vi "04Foot.vi"() -> ()   [LabVIEW 2015]
uses:
  <vilib>/Instr/_visa.llb/VISA Configure Serial Port (Serial Instr).vi
  <vilib>/Utility/file.llb/Read Delimited Spreadsheet (DBL).vi
  <vilib>/DAQmx/create/channels.llb/DAQmx Create Channel (DI-Digital Input).vi
  <vilib>/DAQmx/configure/timing.llb/DAQmx Timing (Sample Clock).vi
  <vilib>/Utility/file.llb/Write Delimited Spreadsheet (DBL).vi
  <resource>/objmgr/daqmx.rc
panel:
  out "MPH READ 2":u8
  in  "Tab Control":enum32{"Page 1", "Page 2"}(tab)
  out "NEXT DURATION":dbl format="%#.1f"
  out "NEXT MPH":dbl min=0.0 max=12.0 step=0.1 format="%.1f"
  out "Time Left":dbl format="%#.0f"
  out "ESTOP":bool
  in  "ESTOP RESUME":bool
  out "MPH":dbl min=0.0 max=12.0 step=0.1 format="%.1f"
  out "Foot":dbl
  out "ESTOP2":bool
  out "Report Location":path
  in  "TestScript":path=path "C:/LabVIEW VIs/TRMConsole/FootTime.txt"
  out "Waveform Graph":dbl[](graph)
  out "speed":dbl[](array[numeric])
  out "time":dbl[](array[numeric])
  out "dwell":dbl[](array[numeric])
  out "step":i32
  out "arraysize":i32
  out "x-y":u32
  out "appended path":path
  out "stopping":bool
  out "String":string
  in  "stop":bool
  out "MPH READ":u8
  in  "Serial Port":refnum<visa-resource-name>="COM8"
  in  "lines":tag="DAQMod1/port0"
  out "Enum":T1(ring)
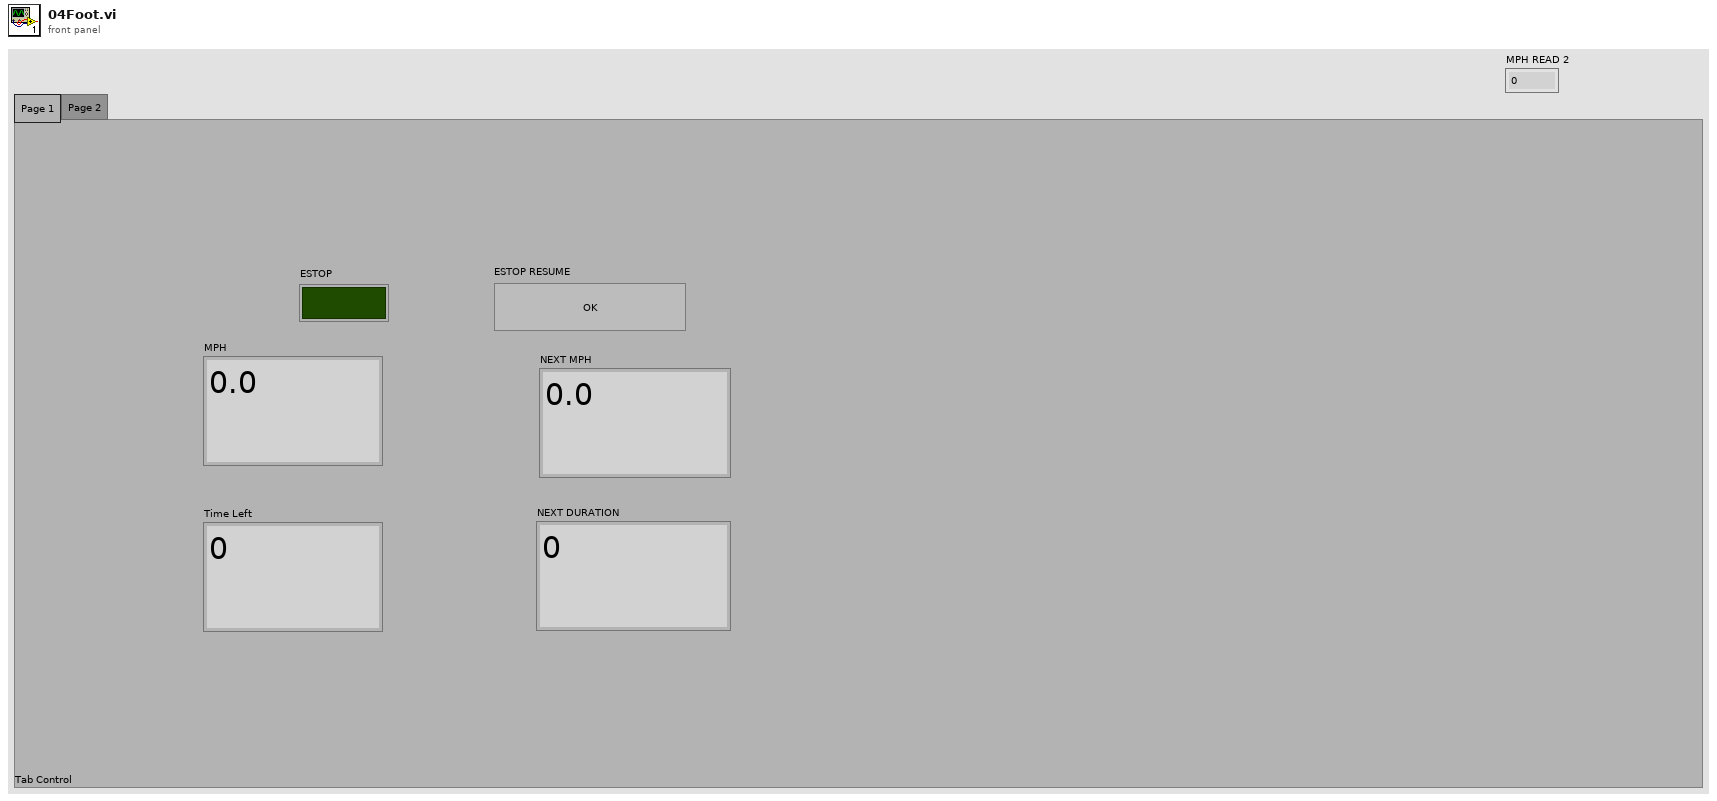
[diagram p1: front panel]
types:
  T1 = enum16{"Initialize", "SetMPH", "GetData", "CheckTiming", "CompressWave", "StartDAQ", "StopDAQ", "Dwell", "WaitforMPH", "ESTOP Wait", "ESTOP Resume"}
  T2 = enum16{"Initialize", "SetMPH", "GetData", "CheckTiming", "CompressWave", "StartDAQ", "StopDAQ", "Dwell", "WaitforMPH"}
  T3 = enum16{"Initialize", "SetMPH", "GetData", "CheckTiming", "CompressWave", "StartDAQ"}
  T4 = enum16{"Initialize", "SetMPH", "GetData", "CheckTiming", "CompressWave"}
  T5 = enum16{"Initialize", "SetMPH", "GetData", "CheckTiming", "CompressWave", "StartDAQ", "StopDAQ"}
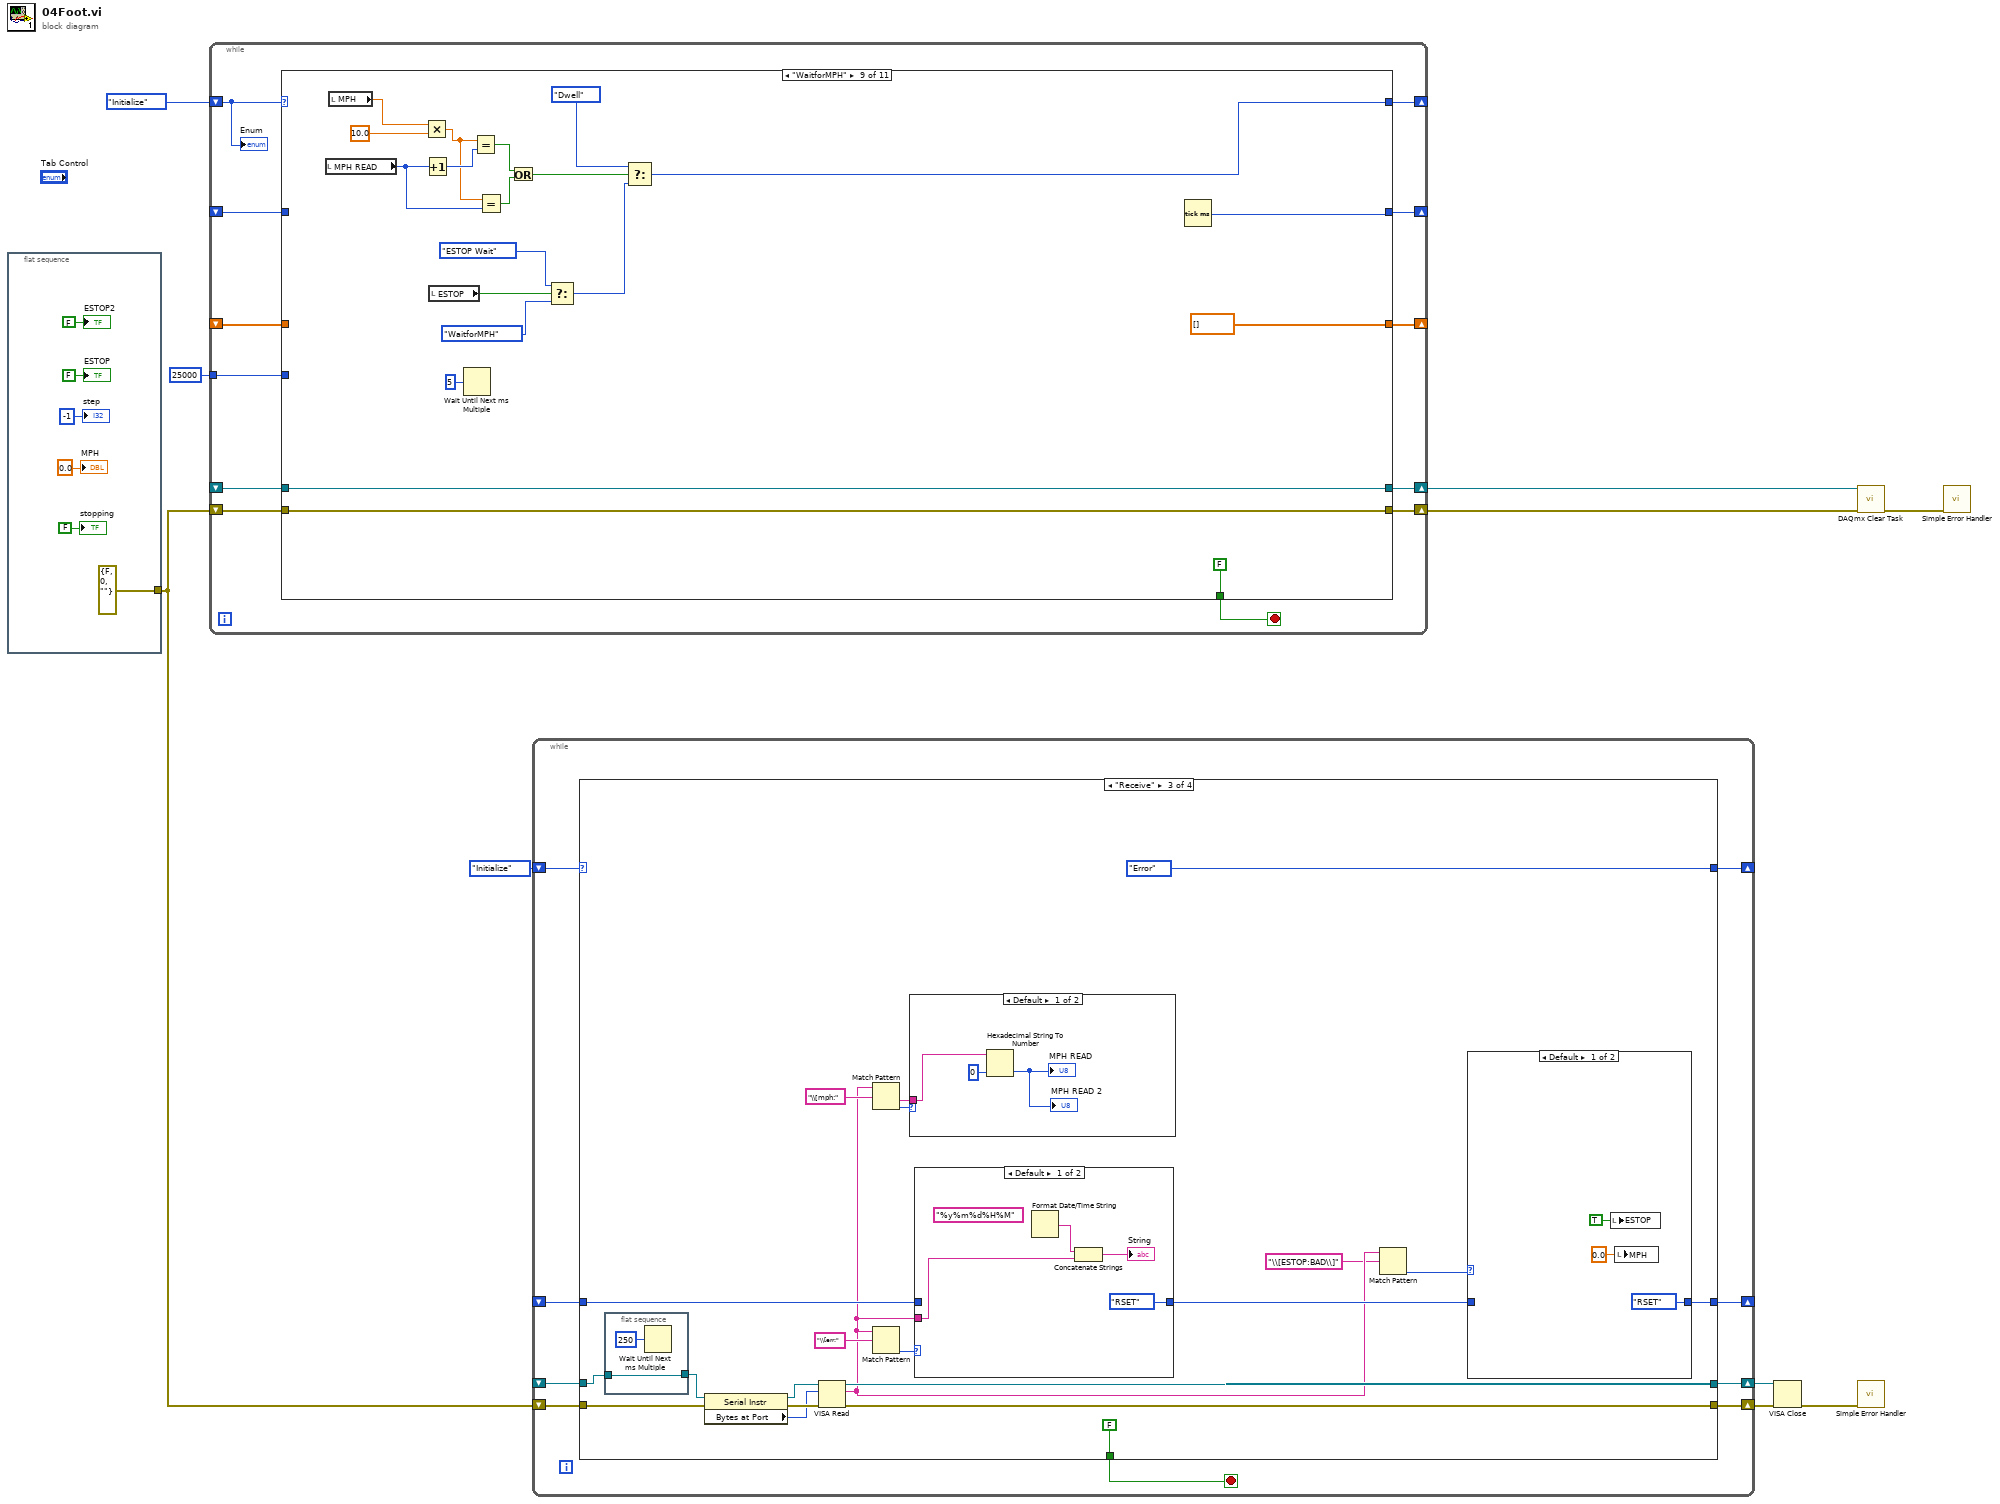
[diagram p0: block diagram]
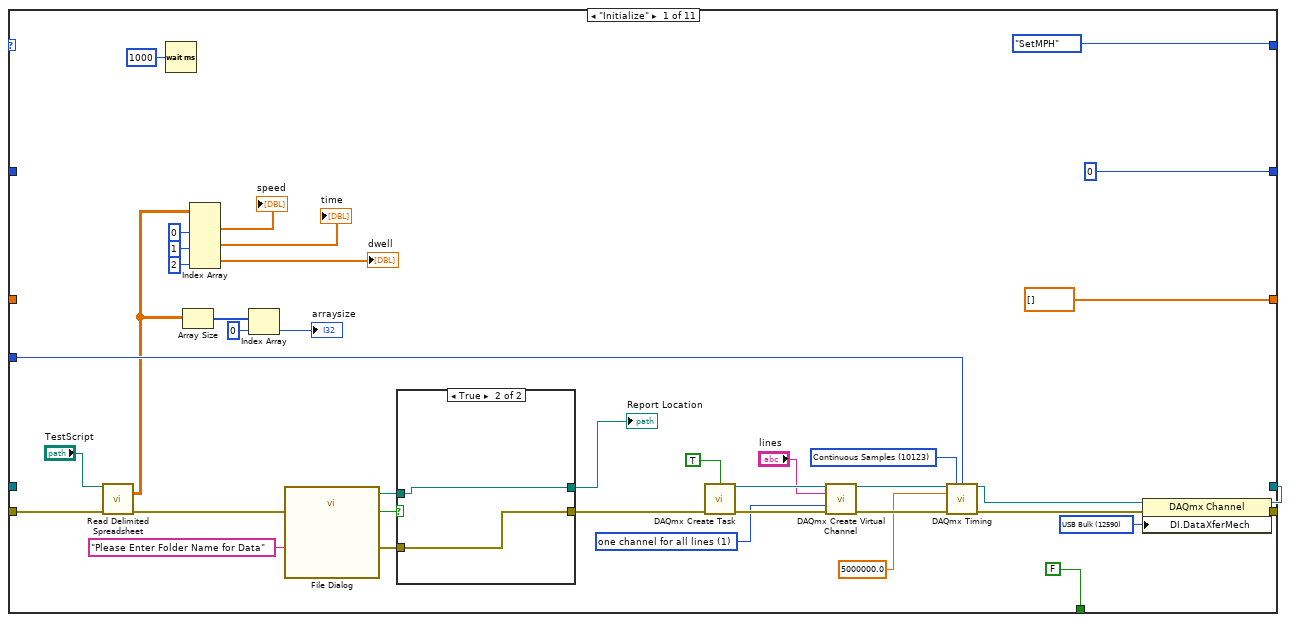
[diagram p2: hidden frame]
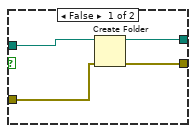
[diagram p3: hidden frame]
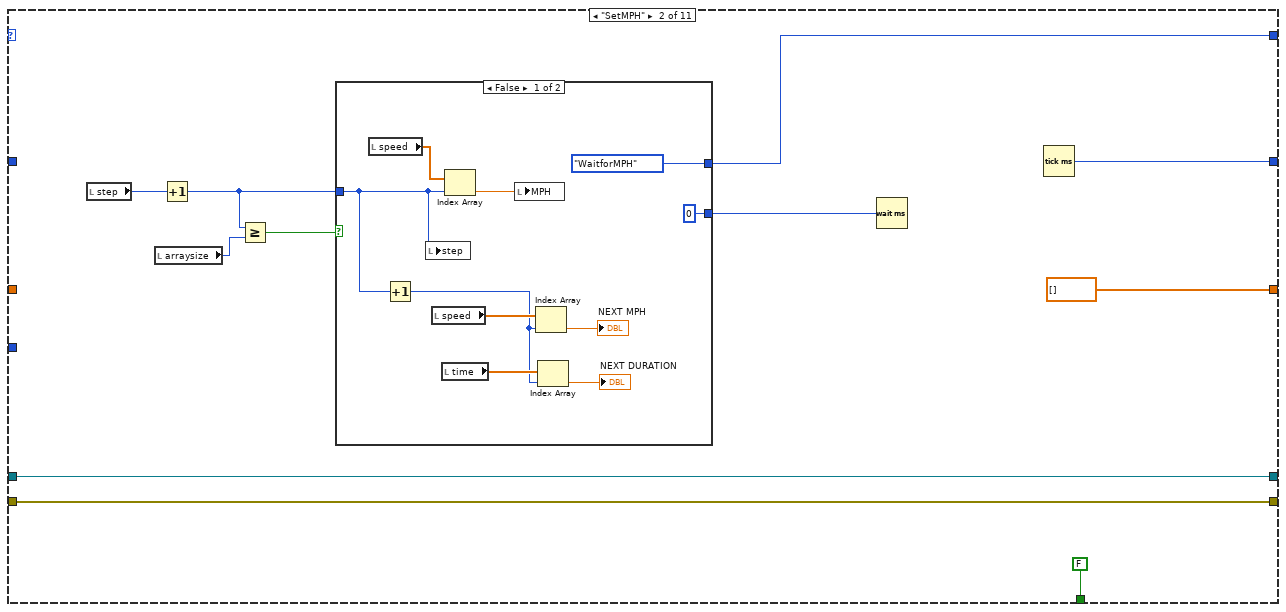
[diagram p4: hidden frame]
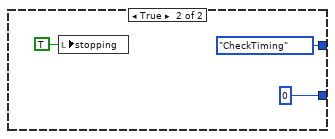
[diagram p5: hidden frame]
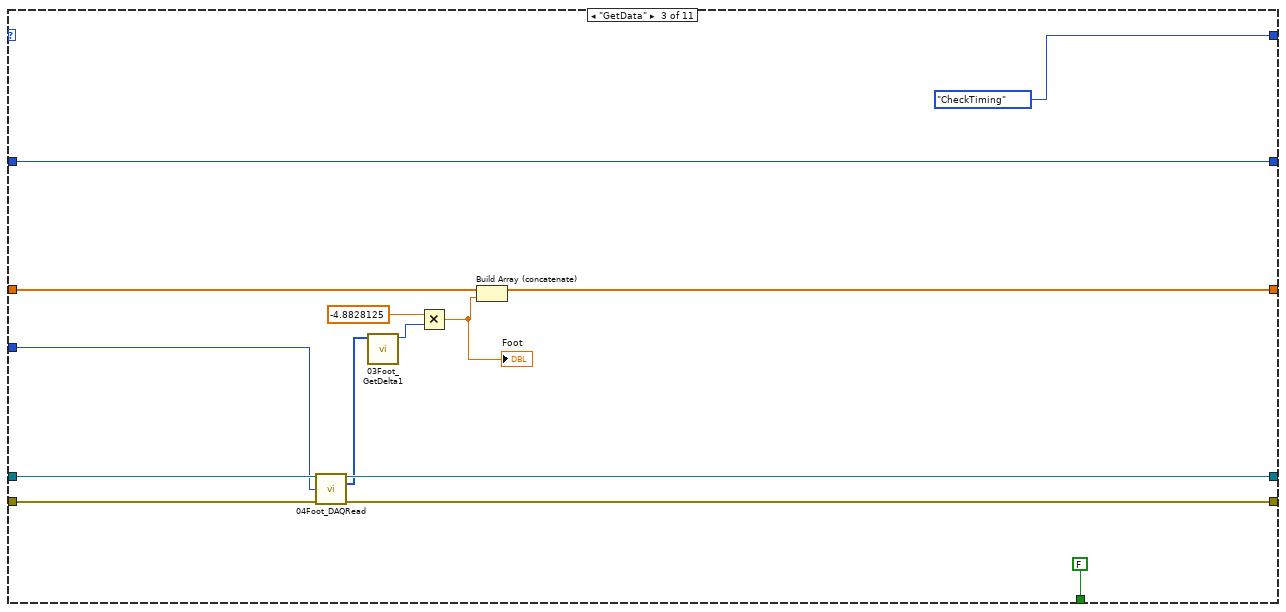
[diagram p6: hidden frame]
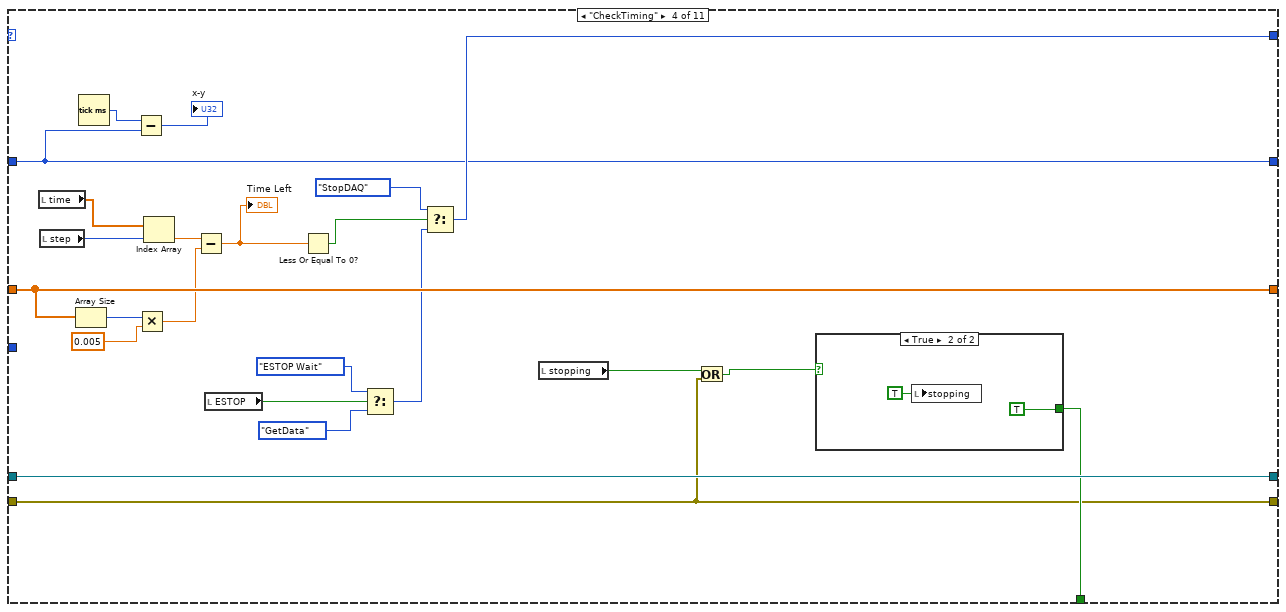
[diagram p7: hidden frame]
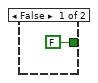
[diagram p8: hidden frame]
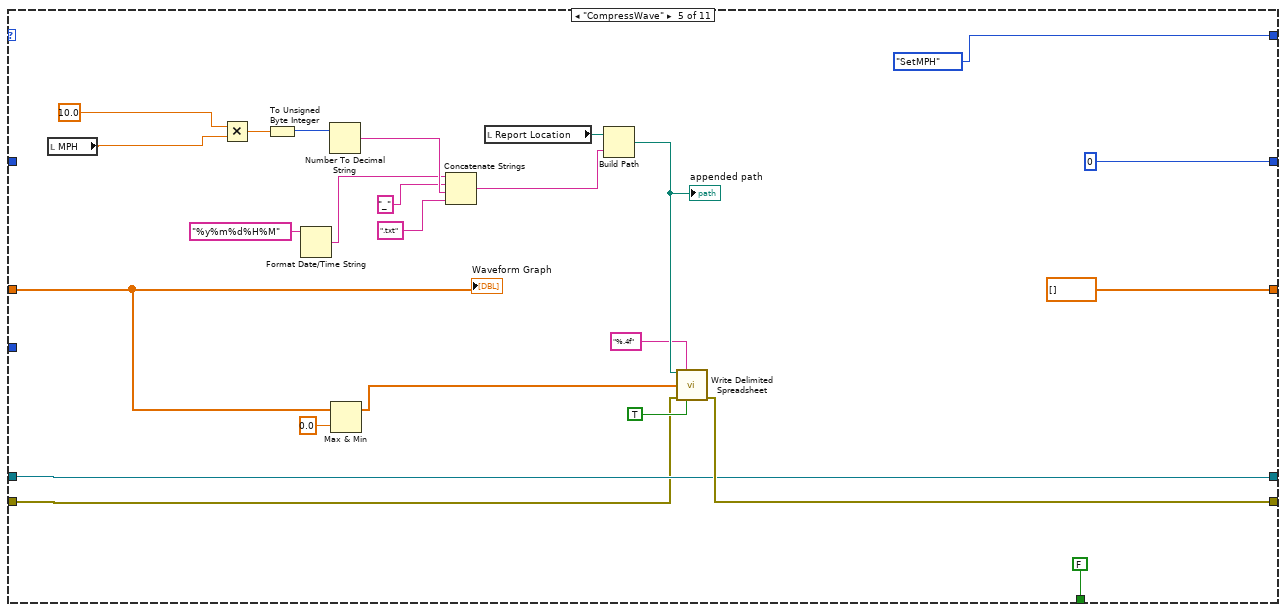
[diagram p9: hidden frame]
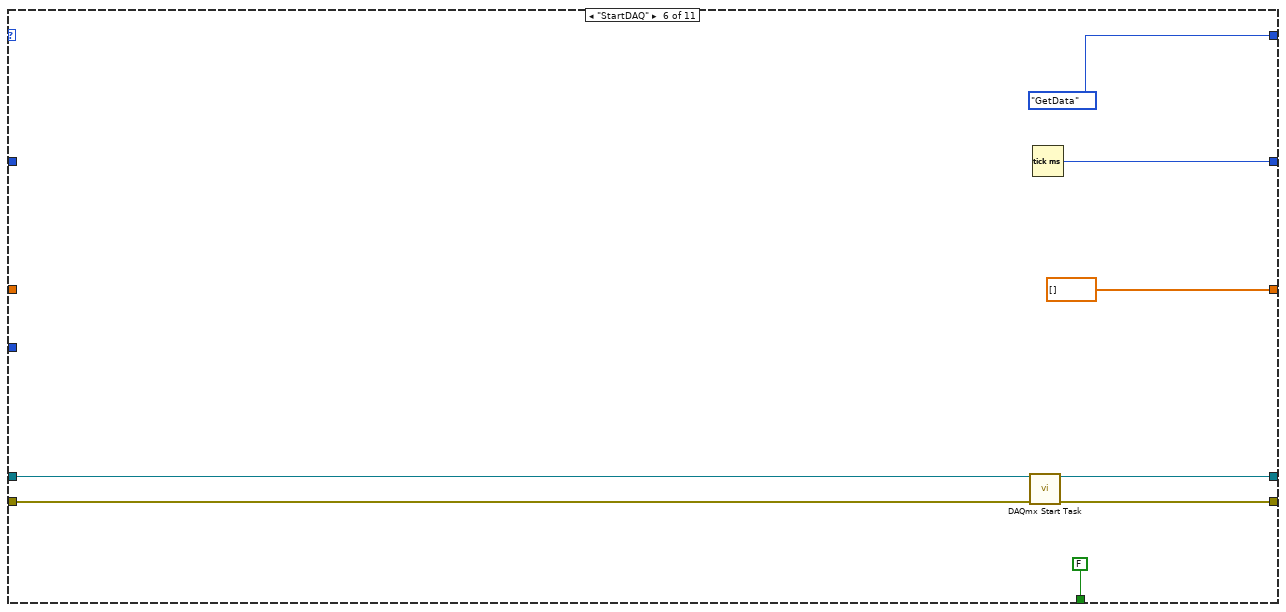
[diagram p10: hidden frame]
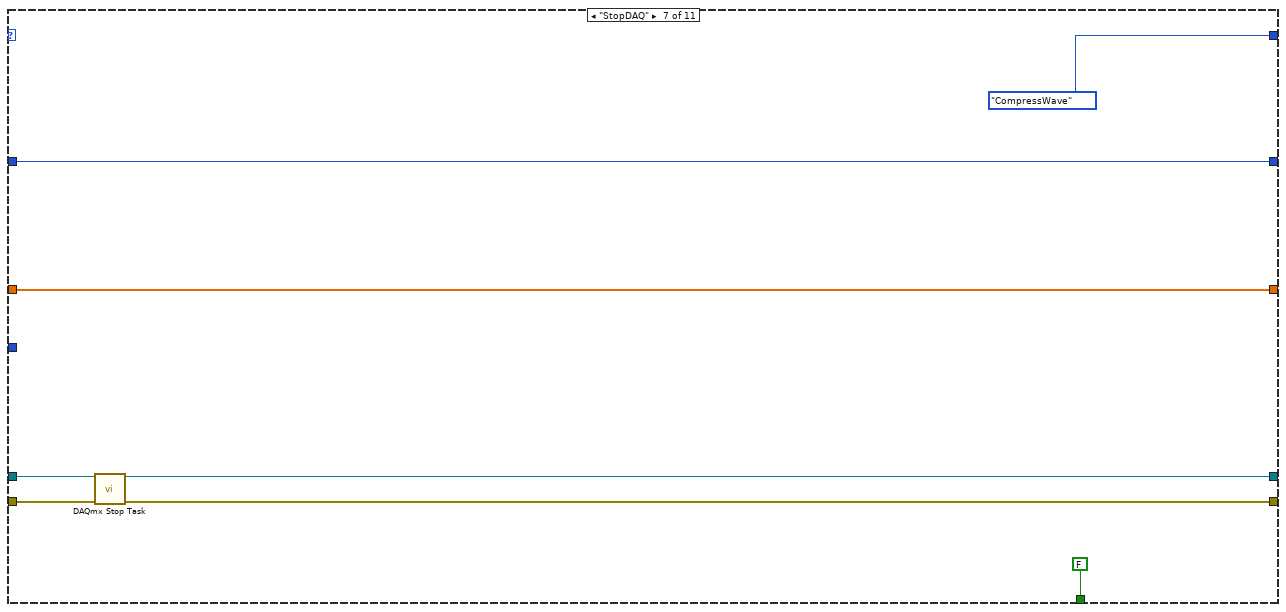
[diagram p11: hidden frame]
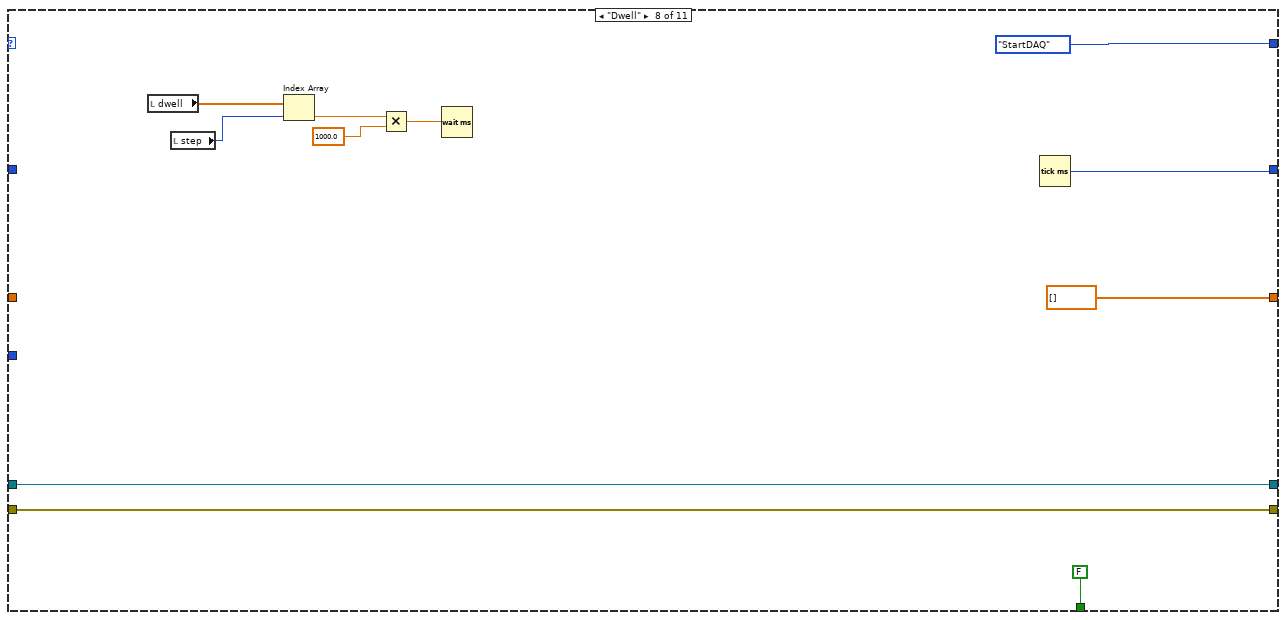
[diagram p12: hidden frame]
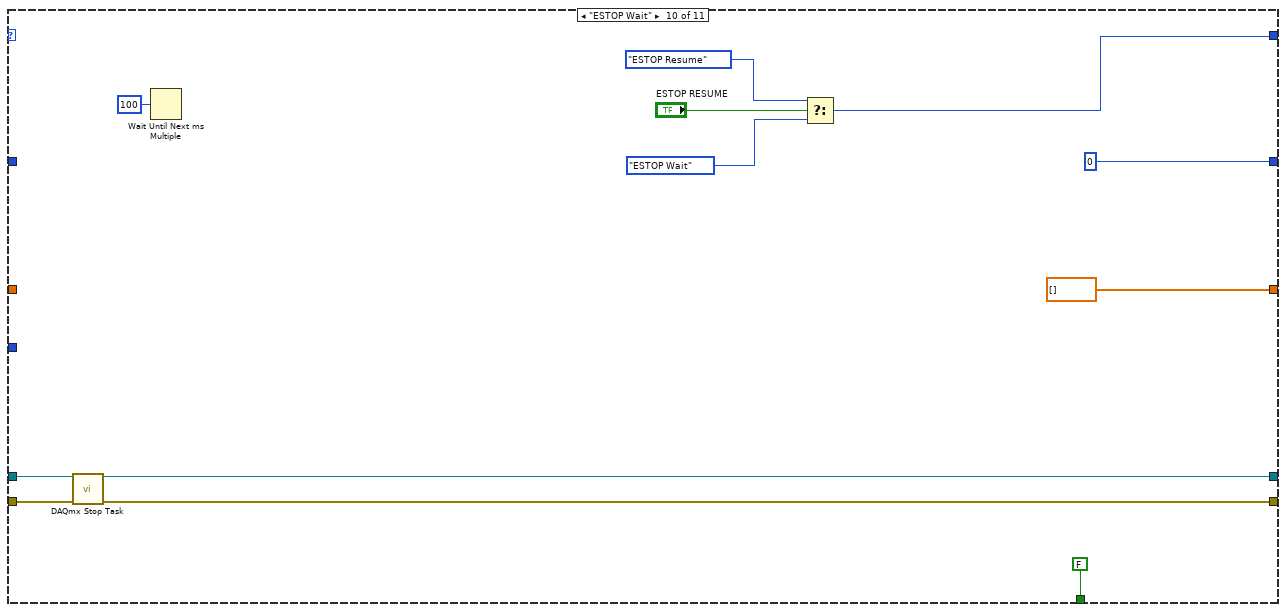
[diagram p13: hidden frame]
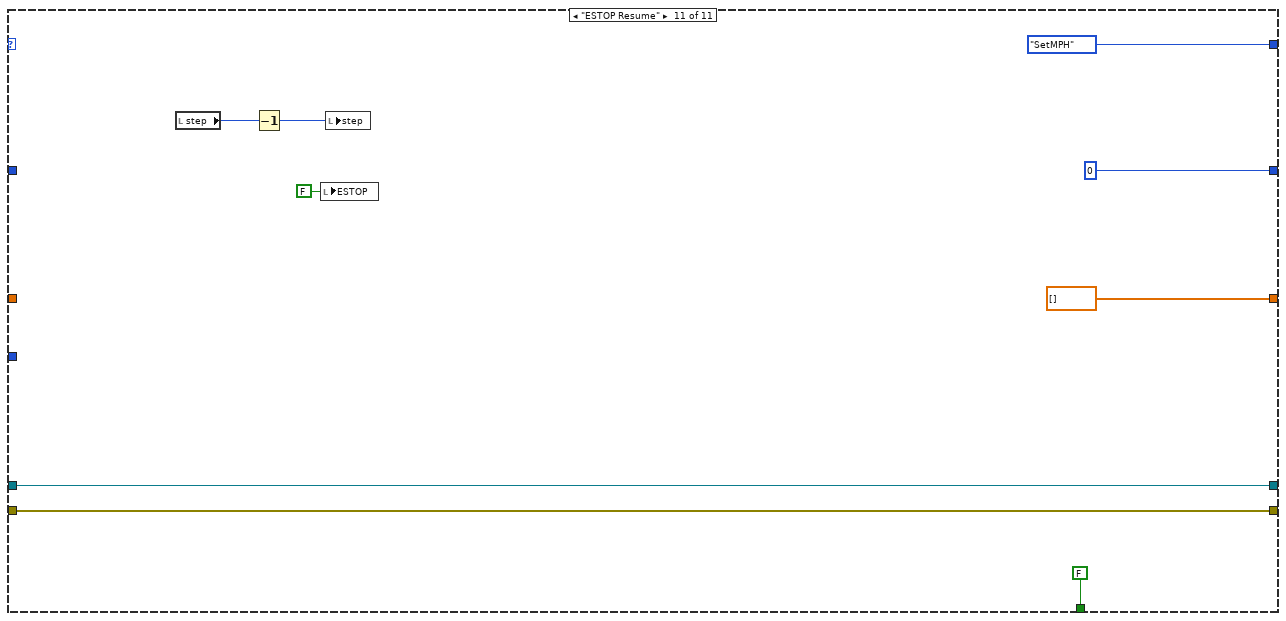
[diagram p14: hidden frame]
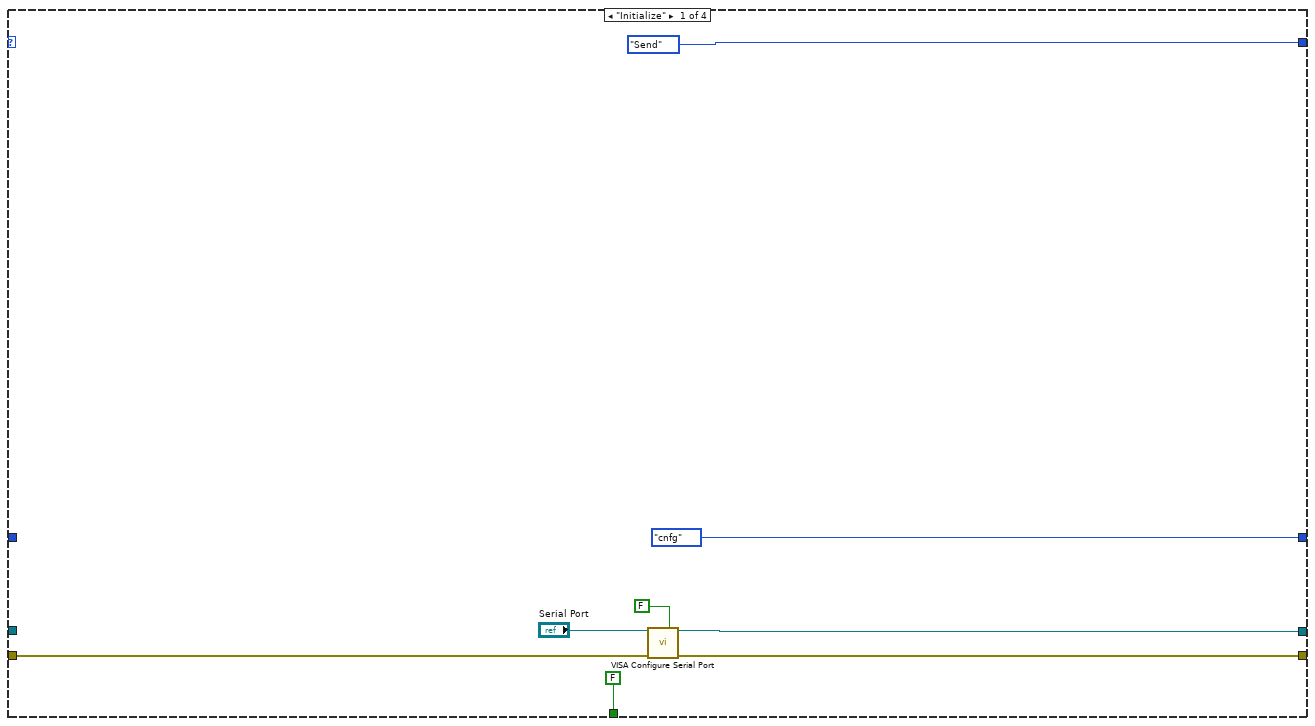
[diagram p15: hidden frame]
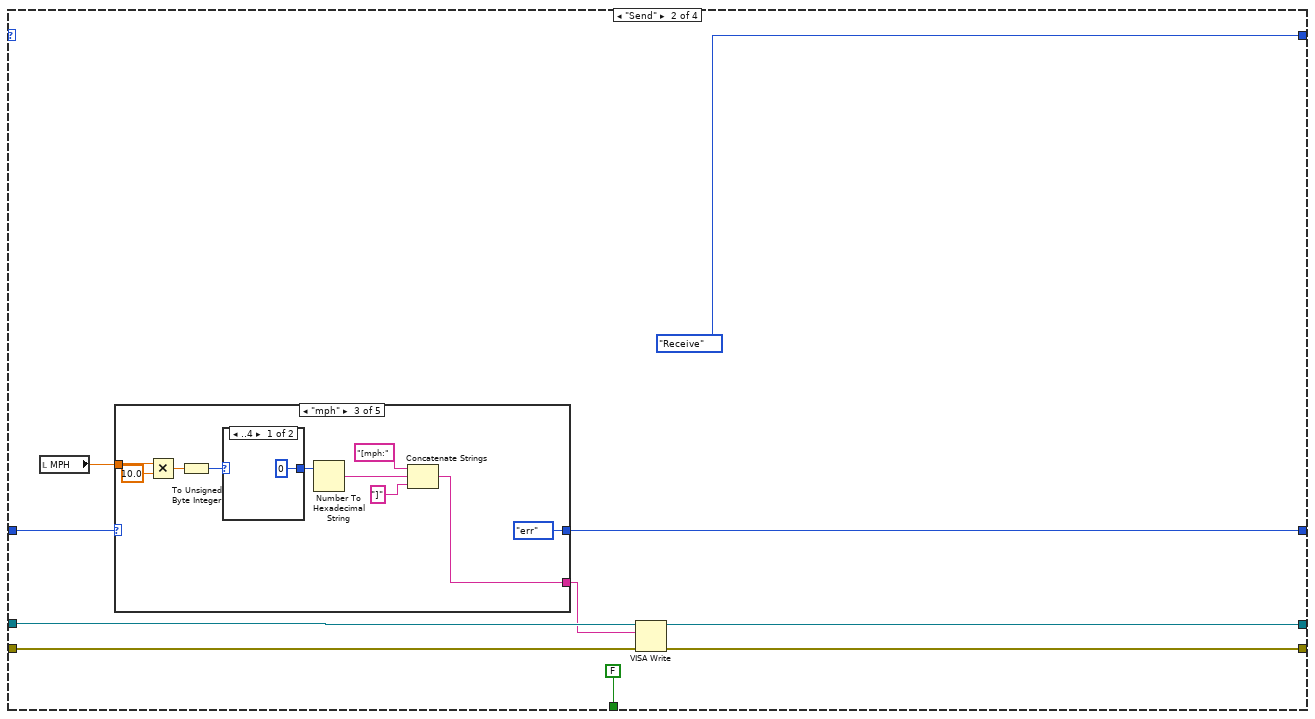
[diagram p16: hidden frame]
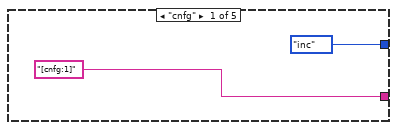
[diagram p17: hidden frame]
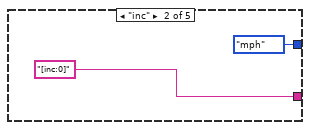
[diagram p18: hidden frame]
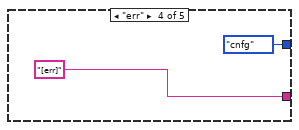
[diagram p20: hidden frame]
diagram:
  n1 = flat-sequence {
    tunnel: [errorcluster {"status"=FALSE, "code"=0, "source"=""} ("error constant")] -> w2
    frame #0 {
      "stopping" <- FALSE ("stopping")
      "MPH" <- 0.0 ("MPH")
      "step" <- -1 ("step")
      "ESTOP" <- FALSE ("ESTOP")
      "ESTOP2" <- FALSE ("ESTOP2")
    }
  }
  n2 = while {
    shift-right: [w28] -> _
    shift-left: T1."Initialize" -> [w17]
    shift-right: [w26] -> w4
    shift-left: _ -> [w24]
    shift-right: [w25] -> w5
    shift-left: w2 -> [w23]
    shift-right: [w22] -> _
    shift-left: _ -> [w21]
    tunnel: 25000 ("samples per channel") -> [w20]
    shift-right: [w19] -> _
    shift-left: _ -> [w18]
    stop <- w27 stop-if-true
    n3 = case shown="\"WaitforMPH\"" w17 {
      tunnel: [T1."SetMPH" w78 T4."CheckTiming" w128 T1."SetMPH" T3."GetData" T5."CompressWave" T2."StartDAQ" w200 w215 T1."SetMPH" ("f")] -> w28
      tunnel: [FALSE FALSE FALSE w132 FALSE FALSE FALSE FALSE FALSE FALSE FALSE] -> w27
      tunnel: [w31 w81 w104 w134 w145 w164 w173 w186 w206 w210 w223] -> w26
      tunnel: [w30 w80 w103 w129 w158 w165 w172 w185 w205 w209 w224] -> w25
      tunnel: w24 -> [_ w81 w106 w134 w145 w163 w175 w186 w206 w212 w223]
      tunnel: w23 -> [w58 w80 w105 w129 w144 w162 w174 w185 w205 w211 w224]
      tunnel: [u32 0 w79 w110 w112 u32 0 w168 w170 w188 w208 u32 0 ("millisecond timer value") u32 0 ("millisecond timer value")] -> w22
      tunnel: w21 -> [_ _ w110 w112 _ _ w170 _ _ _ _]
      tunnel: w20 -> [w55 _ w102 _ _ _ _ _ _ _ _]
      tunnel: [dbl[] [] dbl[] [] w109 w127 dbl[] [] dbl[] [] w176 dbl[] [] dbl[] [] dbl[] [] dbl[] []] -> w19
      tunnel: w18 -> [_ _ w108 w127 w139 _ w176 _ _ _ _]
      frame "Initialize" {
        w29 = 12590 items=["DMA"=10054, "Interrupts"=10204, "Programmed I/O"=10264, "USB Bulk"=12590] ("DI.DataXferMech")
        w54 = 10123 items=["Finite Samples"=10178, "Continuous Samples"=10123, "Hardware Timed Single Point"=12522] ("sample mode")
        w65 = 1 items=["one channel for each line", "one channel for all lines"] ("line grouping")
        n4 = call-poly <vilib>:"Read Delimited Spreadsheet.vi"("file path (dialog if empty)"="TestScript", "error in (no error)"=w58) -> ("all rows"=w43:dbl[][], "error out"=w41:errorcluster)  [unwired: 8 in, 4 out]
        n5 = Wait (ms)(milliseconds to wait=u32 1000) -> ()  [unwired: 1 out]
        n6 = Array Size(array=w43) -> (size(s)=w46:i32[])
        n7 = Index Array(array=w43, index (col) #1=0 ("disabled index (col)"), index (col) #2=1 ("index (col)"), index (col) #3=2 ("index (col)")) -> (element #1=→"speed":dbl[], element #2=→"time":dbl[], element #3=→"dwell":dbl[])  [unwired: 3 in]
        n8 = Index Array(array=w46, index=0) -> (element=→"arraysize":i32)
        n9 = call "File Dialog"("prompt"="Please Enter Folder Name for Data", "error in"=w41) -> ("selected path"=w37:path, "exists"=w39:bool, "error out"=w38:errorcluster)  [unwired: 10 in, 1 out]
        n10 = case shown="True" w39 {
          tunnel: w38 -> [w71 w72]
          tunnel: w37 -> [w70 w73]
          tunnel: [w69 w72] -> w36
          tunnel: [w68 w73] -> w35
          frame False {
            n11 = Create Folder(path (use dialog)=w70, error in=w71) -> (created path=w68:path, error out=w69:errorcluster)  [unwired: 1 in, 1 out]
          }
          frame True {
          }
        }
        "Report Location" <- w35
        n12 = call <vilib>:"DAQmx Create Task.vi"("auto cleanup"=TRUE, "error in"=w36) -> ("task out"=w67:refnum<k21>, "error out"=w66:errorcluster)  [unwired: 12 in]
        n13 = call-poly <vilib>:"DAQmx Create Virtual Channel.vi"("task in"=w67, "lines"="lines", "line grouping"=w65, "error in"=w66) -> ("task out"=w56:refnum<k21>, "error out"=w57:errorcluster)  [unwired: 10 in]
        n14 = call-poly <vilib>:"DAQmx Timing.vi"("task/channels in"=w56, "sample mode"=w54, "samples per channel"=w55, "rate"=5000000.0, "error in"=w57) -> ("task out"=w33:refnum<k21>, "error out"=w32:errorcluster)  [unwired: 9 in]
        n15 = property class="DAQmx Channel"(reference=w33, error in=w32, "DI.DataXferMech"=w29) -> (reference out=w31:refnum<k21>, error out=w30:errorcluster)
      }
      frame "SetMPH" {
        n16 = local read "step"() -> (w75:i32)
        n17 = local read "arraysize"() -> (w77:i32)
        n18 = Increment(x=w75) -> (x+1=w74:i32)
        n19 = Greater Or Equal?(x=w74, y=w77) -> (x >= y?=w76:bool)
        n20 = case shown="False" w76 {
          tunnel: [u32 0 ("milliseconds to wait") u32 0 ("milliseconds to wait")] -> w83
          tunnel: [T2."WaitforMPH" T3."CheckTiming"] -> w78
          tunnel: w74 -> [w90 _]
          frame False {
            n21 = local read "speed"() -> (w93:dbl[])
            n22 = Increment(x=w90) -> (x+1=w85:i32)
            n23 = local write "step"(w90) -> ()
            n24 = local read "speed"() -> (w89:dbl[])
            n25 = local read "time"() -> (w86:dbl[])
            n26 = Index Array(array=w93, index=w90) -> (element=w92:dbl)
            n27 = local write "MPH"(w92) -> ()
            n28 = Index Array(array=w89, index=w85) -> (element=→"NEXT MPH":dbl)
            n29 = Index Array(array=w86, index=w85) -> (element=→"NEXT DURATION":dbl)
          }
          frame True {
            n30 = local write "stopping"(TRUE ("stopping")) -> ()
          }
        }
        n31 = Wait (ms)(milliseconds to wait=w83) -> ()  [unwired: 1 out]
        n32 = Tick Count (ms)() -> (millisecond timer value=w79:u32)
      }
      frame "GetData" {
        n33 = call "04Foot_DAQRead.vi"("task/channels in"=w106, "number of samples per channel"=w102, "error in"=w105) -> ("task out"=w104:refnum<k21>, "data"=w101:u8[], "error out"=w103:errorcluster)  [unwired: 10 in]
        n34 = call "03Foot_GetDelta1.vi"("Array"=w101) -> ("Wave1 Data"=w100:i32)  [unwired: 10 in]
        n35 = Multiply(x=-4.8828125, y=w100) -> (x*y=w98:dbl)
        "Foot" <- w98
        n36 = Build Array (concatenate)(w108, w98) -> (w109:dbl[])
      }
      frame "CheckTiming" {
        n37 = local read "time"() -> (w124:dbl[])
        n38 = local read "step"() -> (w123:i32)
        n39 = Array Size(array=w127) -> (size(s)=w126:i32)
        n40 = Tick Count (ms)() -> (millisecond timer value=w113:u32)
        n41 = Subtract(x=w113, y=w112) -> (x-y=→"x-y":u32)
        n42 = Multiply(x=w126, y=0.005) -> (x*y=w116:dbl)
        n43 = Index Array(array=w124, index=w123) -> (element=w117:dbl)
        n44 = Subtract(x=w117, y=w116) -> (x-y=w115:dbl)
        "Time Left" <- w115
        n45 = local read "ESTOP"() -> (w120:bool)
        n46 = Less Or Equal To 0?(x=w115) -> (x <= 0?=w114:bool)
        n47 = Select(t=T1."ESTOP Wait", s=w120, f=T1."GetData") -> (s? t:f=w118:T1)
        n48 = Select(t=T1."StopDAQ", s=w114, f=w118) -> (s? t:f=w128:T1)
        n49 = local read "stopping"() -> (w131:bool)
        n50 = Or(x=w131, y=w129) -> (x .or. y?=w130:bool)
        n51 = case shown="True" w130 {
          tunnel: [FALSE TRUE] -> w132
          frame False {
          }
          frame True {
            n52 = local write "stopping"(TRUE ("stopping")) -> ()
          }
        }
      }
      frame "CompressWave" {
        n53 = local read "MPH"() -> (w148:dbl)
        n54 = Multiply(x=10.0, y=w148) -> (x*y=w151:dbl)
        n55 = To Unsigned Byte Integer(number=w151) -> (unsigned 8bit integer=w150:u8)
        n56 = Format Date/Time String(time format string (%c)="%y%m%d%H%M") -> (date/time string=w140:string)  [unwired: 2 in]
        n57 = Number To Decimal String(number=w150) -> (decimal integer string=w149:string)  [unwired: 1 in]
        n58 = Max & Min(x=w139, y=0.0) -> (max(x,y)=w146:dbl[])  [unwired: 1 out]
        n59 = Concatenate Strings(w140, "_" ("string"), w149, ".txt" ("string")) -> (w154:string)
        n60 = local read "Report Location"() -> (w143:path)
        n61 = Build Path(base path=w143, name or relative path=w154) -> (appended path=w153:path)
        "appended path" <- w153
        n62 = call-poly <vilib>:"Write Delimited Spreadsheet.vi"("file path (dialog if empty)"=w153, "format (%.3f)"="%.4f", "1D data"=w146, "error in (no error)"=w144, "transpose? (F)"=TRUE) -> ("error out"=w158:errorcluster)  [unwired: 9 in, 1 out]
        "Waveform Graph" <- w139
      }
      frame "StartDAQ" {
        n63 = call <vilib>:"DAQmx Start Task.vi"("task/channels in"=w163, "error in"=w162) -> ("task out"=w164:refnum<k21>, "error out"=w165:errorcluster)  [unwired: 12 in]
        n64 = Tick Count (ms)() -> (millisecond timer value=w168:u32)
      }
      frame "StopDAQ" {
        n65 = call <vilib>:"DAQmx Stop Task.vi"("task/channels in"=w175, "error in"=w174) -> ("task out"=w173:refnum<k21>, "error out"=w172:errorcluster)  [unwired: 12 in]
      }
      frame "Dwell" {
        n66 = local read "dwell"() -> (w183:dbl[])
        n67 = local read "step"() -> (w182:i32)
        n68 = Index Array(array=w183, index=w182) -> (element=w181:dbl)
        n69 = Multiply(x=w181, y=1000.0) -> (x*y=w179:dbl)
        n70 = Wait (ms)(milliseconds to wait=w179) -> ()  [unwired: 1 out]
        n71 = Tick Count (ms)() -> (millisecond timer value=w188:u32)
      }
      frame "WaitforMPH" {
        n72 = local read "MPH READ"() -> (w192:u8)
        n73 = local read "MPH"() -> (w203:dbl)
        n74 = Multiply(x=w203, y=10.0) -> (x*y=w193:dbl)
        n75 = Increment(x=w192) -> (x+1=w201:u8)
        n76 = local read "ESTOP"() -> (w198:bool)
        n77 = Wait Until Next ms Multiple(millisecond multiple=u32 5) -> ()  [unwired: 1 out]
        n78 = Equal?(x=w193, y=w201) -> (x = y?=w190:bool)
        n79 = Equal?(x=w193, y=w192) -> (x = y?=w191:bool)
        n80 = Or(x=w190, y=w191) -> (x .or. y?=w189:bool)
        n81 = Select(t=T1."ESTOP Wait", s=w198, f=T1."WaitforMPH") -> (s? t:f=w195:T1)
        n82 = Select(t=T1."Dwell", s=w189, f=w195) -> (s? t:f=w200:T1)
        n83 = Tick Count (ms)() -> (millisecond timer value=w208:u32)
      }
      frame "ESTOP Wait" {
        n84 = call <vilib>:"DAQmx Stop Task.vi"("task/channels in"=w212, "error in"=w211) -> ("task out"=w210:refnum<k21>, "error out"=w209:errorcluster)  [unwired: 12 in]
        n85 = Wait Until Next ms Multiple(millisecond multiple=u32 100) -> ()  [unwired: 1 out]
        n86 = Select(t=T1."ESTOP Resume", s="ESTOP RESUME", f=T1."ESTOP Wait") -> (s? t:f=w215:T1)
      }
      frame "ESTOP Resume" {
        n87 = local read "step"() -> (w229:i32)
        n88 = Decrement(x=w229) -> (x-1=w228:i32)
        n89 = local write "ESTOP"(FALSE ("ESTOP")) -> ()
        n90 = local write "step"(w228) -> ()
      }
    }
    "Enum" <- w17
  }
  n91 = while {
    shift-right: [w234] -> w8
    shift-left: w2 -> [w238]
    shift-right: [w235] -> w9
    shift-left: _ -> [w237]
    shift-right: [w233] -> _
    shift-left: enum16{"Initialize", "Send", "Receive", "Error"}."Initialize" -> [w236]
    shift-right: [w232] -> _
    shift-left: _ -> [w231]
    stop <- w230 stop-if-true
    n92 = case shown="\"Receive\"" w236 {
      tunnel: w238 -> [w242 w254 w293 w313]
      tunnel: w237 -> [_ w253 w292 w317]
      tunnel: [w244 w256 w291 w317] -> w235
      tunnel: [w243 w255 w285 w313] -> w234
      tunnel: [enum16{"Initialize", "Send", "Receive", "Error"}."Send" enum16{"Initialize", "Send", "Receive", "Error"}."Receive" enum16{"Initialize", "Send", "Receive", "Error"}."Error" enum16{"Initialize", "Send", "Receive", "Error"}."Send"] -> w233
      tunnel: [enum16{"cnfg", "inc", "mph", "err", "RSET"}."cnfg" w250 w279 w318] -> w232
      tunnel: w231 -> [_ w251 w286 w318]
      tunnel: [FALSE FALSE FALSE w312] -> w230
      frame "Initialize" {
        n93 = call-poly "VISA Configure Serial Port"("VISA resource name"="Serial Port", "Enable Termination\nChar (T)"=FALSE ("Enable Termination\nChar (T)"), "error in (no error)"=w242) -> ("VISA resource name out"=w244:refnum<visa-resource-name>, "error out"=w243:errorcluster)  [unwired: 11 in]
      }
      frame "Send" {
        n94 = local read "MPH"() -> (w247:dbl)
        n95 = case shown="\"mph\"" w251 {
          tunnel: ["[cnfg:1]" "[inc:0]" w261 "[err]" "[RSET]"] -> w252
          tunnel: w247 -> [_ _ w270 _ _]
          tunnel: [enum16{"cnfg", "inc", "mph", "err", "RSET"}."inc" enum16{"cnfg", "inc", "mph", "err", "RSET"}."mph" enum16{"cnfg", "inc", "mph", "err", "RSET"}."err" enum16{"cnfg", "inc", "mph", "err", "RSET"}."cnfg" enum16{"cnfg", "inc", "mph", "err", "RSET"}."cnfg"] -> w250
          frame "cnfg" {
          }
          frame "inc" {
          }
          frame "mph" {
            n96 = Multiply(x=w270, y=10.0) -> (x*y=w264:dbl)
            n97 = To Unsigned Byte Integer(number=w264) -> (unsigned 8bit integer=w263:u8)
            n98 = case shown="..4" w263 {
              selector: w263 -> [_ w272]
              tunnel: [u8 0 w272] -> w262
              frame ..4 {
              }
              frame 5.. {
              }
            }
            n99 = Number To Hexadecimal String(2:w262) -> (0:w267:string)  [unwired: 1 in]
            n100 = Concatenate Strings("[mph:" ("string"), w267, "]" ("string")) -> (w261:string)
          }
          frame "err" {
          }
          frame "RSET" {
          }
        }
        n101 = VISA Write(VISA resource name=w253, write buffer=w252, error in (no error)=w254) -> (VISA resource name out=w256:refnum<visa-resource-name>, error out=w255:errorcluster)  [unwired: 1 out]
      }
      frame "Receive" {
        n102 = flat-sequence {
          tunnel: w292 -> [w310]
          tunnel: [w310] -> w297
          frame #0 {
            n103 = Wait Until Next ms Multiple(millisecond multiple=u32 250) -> ()  [unwired: 1 out]
          }
        }
        n104 = property class="Serial Instr"(reference=w297, error in=w293) -> (reference out=w295:refnum<visa-resource-name>, error out=w296:errorcluster, "Bytes at Port"=w294:u32)
        n105 = VISA Read(VISA resource name=w295, byte count=w294, error in (no error)=w296) -> (VISA resource name out=w291:refnum<visa-resource-name>, read buffer=w280:string, error out=w285:errorcluster)  [unwired: 1 out]
        n106 = Match Pattern(string=w280, regular expression="\\[mph:") -> (after substring=w282:string, offset past match=w283:i32)  [unwired: 1 in, 2 out]
        n107 = Match Pattern(string=w280, regular expression="\\[err:") -> (offset past match=w287:i32)  [unwired: 1 in, 3 out]
        n108 = case shown="Default" w283 {
          tunnel: w282 -> [w304 _]
          frame Default {
            n109 = Hexadecimal String To Number(string=w304, default (0uL)=u8 0 ("default (0 I32)")) -> (number=→"MPH READ" →"MPH READ 2":u8)  [unwired: 1 in, 1 out]
          }
          frame -1 {
          }
        }
        n110 = case shown="Default" w287 {
          tunnel: [enum16{"cnfg", "inc", "mph", "err", "RSET"}."RSET" w309] -> w281
          tunnel: w286 -> [_ w309]
          tunnel: w280 -> [w305 _]
          frame Default {
            (unwired) "%y%m%d%H%M" ("time format string (%c)")
            n111 = Format Date/Time String() -> (date/time string=w306:string)  [unwired: 3 in]
            n112 = Concatenate Strings(w306, w305) -> (→"String":string)
          }
          frame -1 {
          }
        }
        n113 = Match Pattern(string=w280, regular expression="\\[ESTOP:BAD\\]") -> (offset past match=w278:i32)  [unwired: 1 in, 3 out]
        n114 = case shown="Default" w278 {
          tunnel: w281 -> [_ w301]
          tunnel: [enum16{"cnfg", "inc", "mph", "err", "RSET"}."RSET" w301] -> w279
          frame Default {
            n115 = local write "ESTOP"(TRUE ("ESTOP")) -> ()
            n116 = local write "MPH"(0.0 ("MPH")) -> ()
          }
          frame -1 {
          }
        }
      }
      frame "Error" {
        n117 = local read "stopping"() -> (w314:bool)
        n118 = Compound Arithmetic op=OR("stop", w314, w313) -> (w316:bool)
        n119 = case shown="True" w316 {
          tunnel: [FALSE TRUE] -> w312
          frame False {
          }
          frame True {
            n120 = local write "stopping"(TRUE ("stopping")) -> ()
          }
        }
      }
    }
  }
  n121 = VISA Close(VISA resource name=w9, error in (no error)=w8) -> (error out=w7:errorcluster)
  n122 = call <vilib>:"DAQmx Clear Task.vi"("task in"=w4, "error in"=w5) -> ("error out"=w3:errorcluster)  [unwired: 13 in]
  n123 = call <vilib>:"Simple Error Handler.vi"("error in (no error)"=w7) -> ()  [unwired: 4 in, 5 out]
  n124 = call <vilib>:"Simple Error Handler.vi"("error in (no error)"=w3) -> ()  [unwired: 4 in, 5 out]
